vi "motion.vi"(11 "A3200.lvclass in":refnum<class "A3200.lvclass">) -> (3 "A3200.lvclass out":refnum<class "A3200.lvclass">)   [LabVIEW 2016]
uses:
  Classes/Controller/Motion/A3200 Folder/A3200.lvclass
panel:
  in  "stop":bool
  in  "Tab Control":enum32{"XYZU JOG", "GO", "controller"}(tab)
  in  "Z go":bool
  in  "XYZU go":bool
  in  "XY go":bool
  in  "XY Position":dbl[](array[numeric])=[600.0, 600.0]
  in  "Z Position":dbl format="%#_13g"
  in  "XY Speed":dbl=50.0
  in  "Z Speed":dbl=20.0
  in  "XYZU Position":dbl[](array[numeric])=[500.0, 500.0, 5.0]
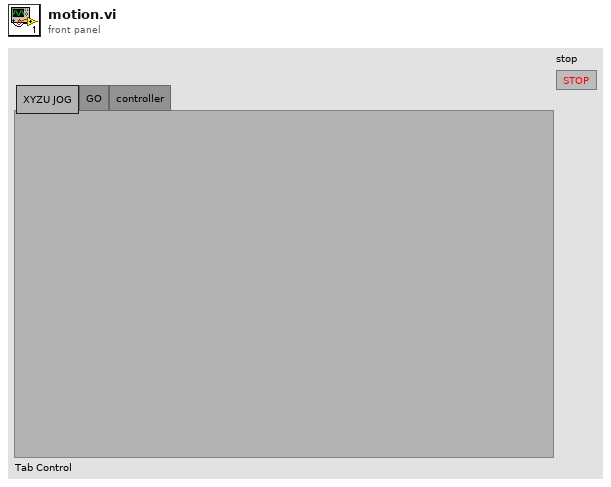
[diagram p1: front panel]
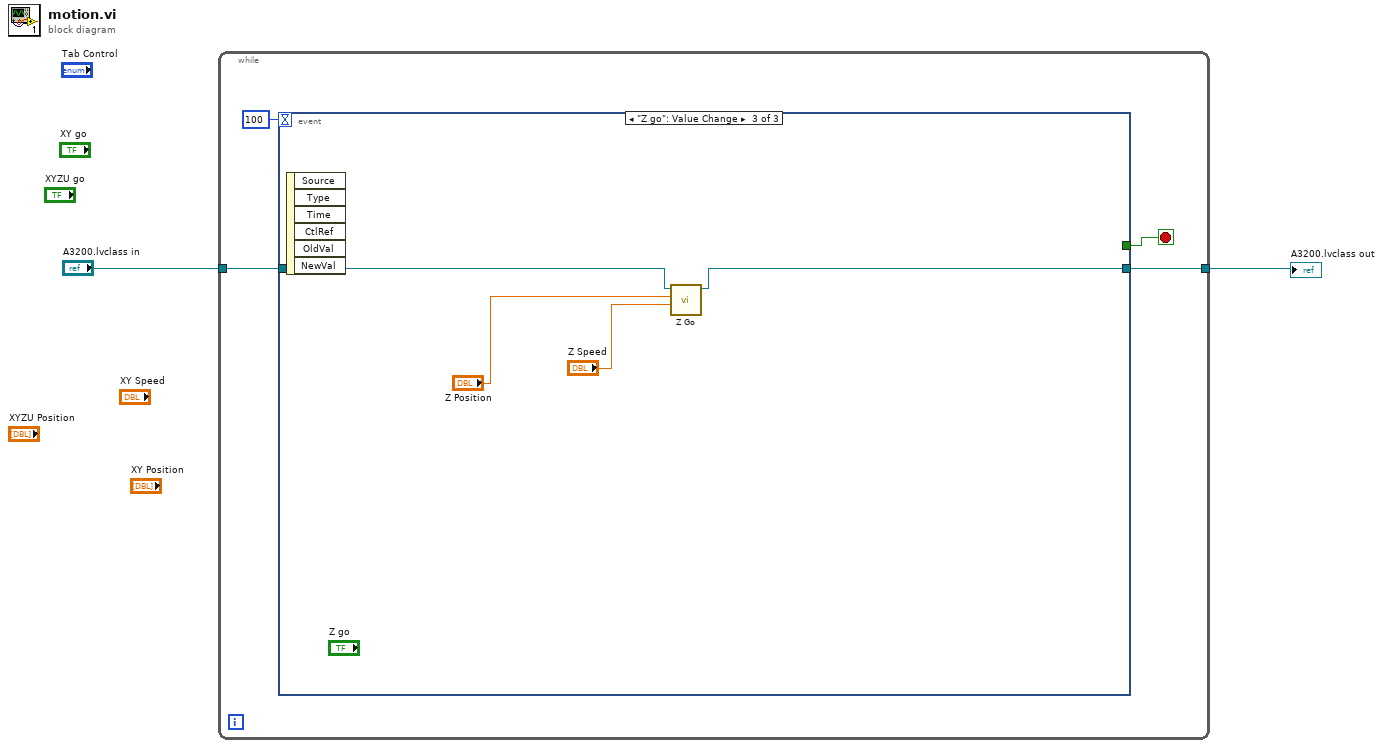
[diagram p0: block diagram]
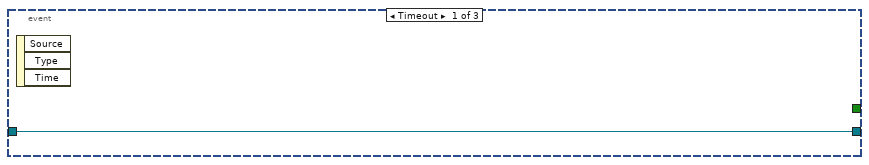
[diagram p2: hidden frame]
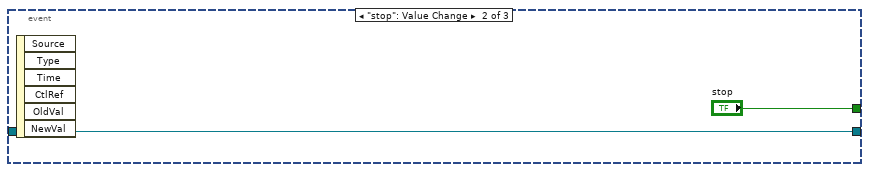
[diagram p3: hidden frame]
diagram:
  n1 = while {
    tunnel: "A3200.lvclass in" -> [w4]
    tunnel: [w3] -> w1
    stop <- w6 stop-if-true
    n2 = event shown="[2] \"Z go\": Value Change" {
      selector: _ -> [_ _ _]
      dyn-events: _ -> [_ _ _]
      timeout: 100 -> [_ _ _]
      tunnel: [_ "stop" _] -> w6
      tunnel: w4 -> [w7 w8 w13]
      tunnel: [w7 w8 w12] -> w3
      event Timeout {
        n3 = event-data() -> ()  [unwired: 1 in, 3 out]
      }
      event "stop": Value Change {
        n4 = event-data() -> ()  [unwired: 1 in, 6 out]
      }
      event "Z go": Value Change {
        n5 = event-data() -> ()  [unwired: 1 in, 6 out]
        n6 = call-dynamic "Z Go.vi"("Speed"="Z Speed", "Position"="Z Position", "Gantry in"=w13) -> ("Gantry out"=w12:refnum<class "A3200.lvclass">)  [unwired: 7 in, 1 out]
      }
    }
  }
  "A3200.lvclass out" <- w1
